vi "Check Path.vi"(2 "path":path) -> (4 "Path String":string)   [LabVIEW 2021, in "CIF Configuration File.lvlib"]
uses:
  CIF Configuration File.lvlib
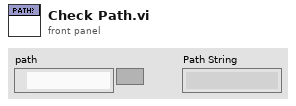
[diagram p1: front panel]
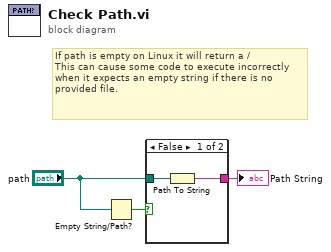
[diagram p0: block diagram]
diagram:
  # "If path is empty on Linux it will return a / \nThis can cause some code to execute incorrectly when it expects an empty string if there is no provided file."
  n1 = Empty String/Path?(string/path="path") -> (empty?=w2:bool)
  n2 = case shown="False" w2 {
    tunnel: "path" -> [w5 _]
    tunnel: [w4 _] -> w1
    frame False {
      n3 = Path To String(path=w5) -> (string=w4:string)
    }
    frame True {
    }
  }
  "Path String" <- w1
